vi "Deadbandv1.vi"(1 "Deadband":cluster{dbl, dbl}, 2 "Value":cluster{dbl, dbl}) -> (0 "Value Out":cluster{dbl, dbl})   [LabVIEW 2013]
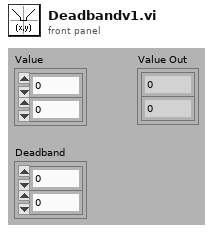
[diagram p1: front panel]
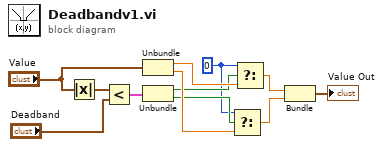
[diagram p0: block diagram]
diagram:
  w1 = 0
  n1 = Absolute Value(x="Value") -> (abs(x)=w12:cluster{dbl, dbl})
  n2 = Less?(x=w12, y="Deadband") -> (x < y?=w5:cluster{bool, bool})
  n3 = Unbundle("Value") -> (w7:dbl, w8:dbl)
  n4 = Unbundle(w5) -> (w3:bool, w4:bool)
  n5 = Select(t=w1, s=w4, f=w8) -> (s? t:f=w10:dbl)
  n6 = Select(t=w1, s=w3, f=w7) -> (s? t:f=w9:dbl)
  n7 = Bundle(w9, w10) -> (→"Value Out":cluster{dbl, dbl})  [unwired: 1 out]
